vi "Update AppInst Ring and Select Project.vi"(8 "error in":errorcluster, 10 "Project Name":string, 11 "Ring in":refnum<vi>) -> (0 "error out":errorcluster, 2 "AppInst out":refnum<vi>)   [LabVIEW 2013, in "LVTM.lvlib"]
uses:
  LVTM.lvlib
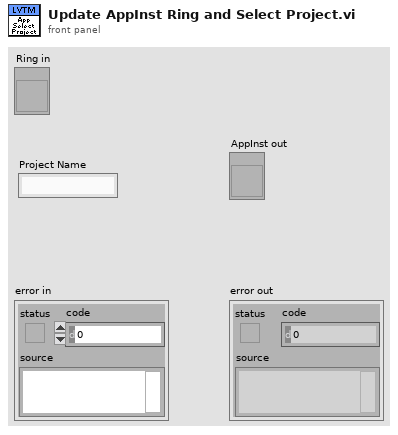
[diagram p1: front panel]
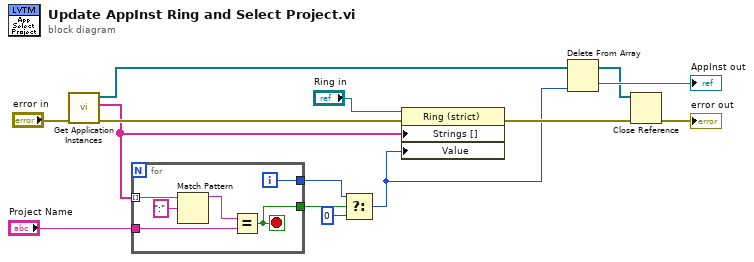
[diagram p0: block diagram]
diagram:
  n1 = call "Get Application Instances.vi"("error in (no error)"="error in") -> ("error out"=w9:errorcluster, "App Instance Names"=w6:string[], "App Instances"=w13:refnum<vi>[])  [unwired: 8 in]
  n2 = for {
    tunnel: w6 -> [w20] mode=indexing
    tunnel: "Project Name" -> [w17]
    tunnel: [w16] -> w3
    tunnel: [w15] -> w4
    i -> [w16]
    stop <- w15 stop-if-true
    n3 = Match Pattern(string=w20, regular expression=":") -> (before substring=w18:string)  [unwired: 1 in, 3 out]
    n4 = Equal?(x=w18, y=w17) -> (x = y?=w15:bool)
  }
  n5 = Select(t=w3, s=w4, f=0) -> (s? t:f=w1:i32)
  n6 = property class="Ring (strict)"(reference="Ring in", error in=w9, "Strings []"=w6, "Value"=w1) -> (error out=w8:errorcluster)  [unwired: 1 out]
  n7 = Delete From Array(array=w13, index=w1) -> (deleted portion=→"AppInst out":refnum<vi>, array with subset deleted=w11:refnum<vi>[])  [unwired: 1 in]
  n8 = Close Reference(reference=w11, error in (no error)=w8) -> (error out=→"error out":errorcluster)
